vi "DoGetNewUser.vi"(8 "error in (no error)":errorcluster, 9 "LastUserName":string, 10 "IsInitialLogin":bool, 11 "Sequence Context In":refnum<k7>) -> (0 "error out":errorcluster, 1 "LoginName":string, 2 "isValidUser":bool, 3 "Sequence Context Out":refnum<k7>, 5 "logOut":bool)   [LabVIEW 2021]
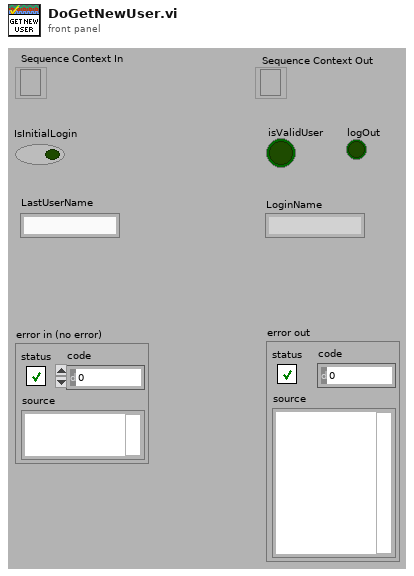
[diagram p1: front panel]
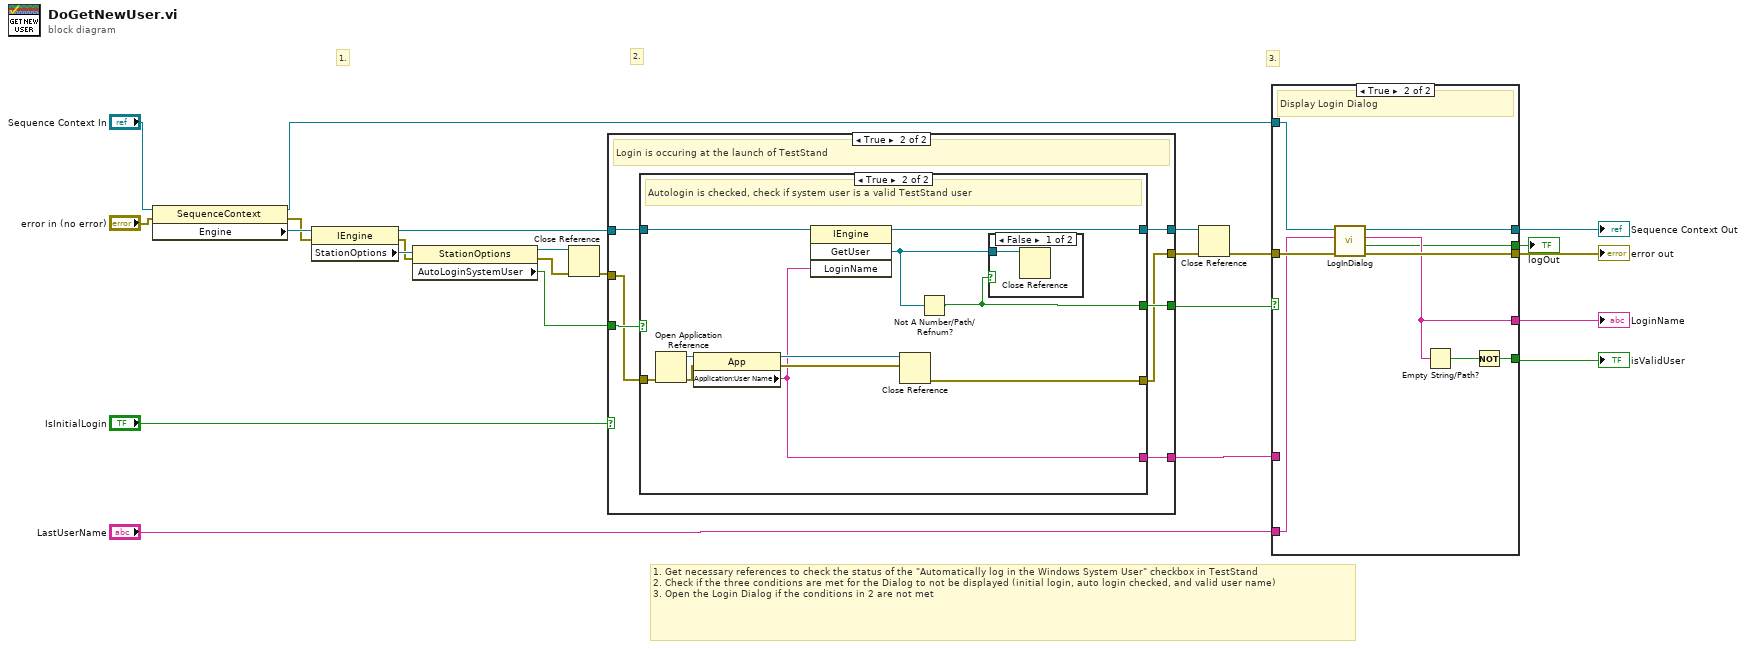
[diagram p0: block diagram]
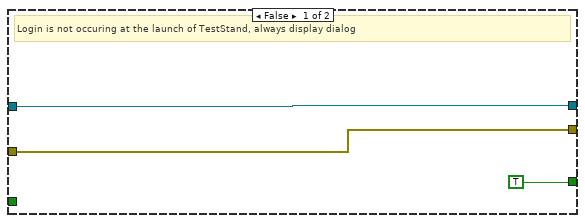
[diagram p2: hidden frame]
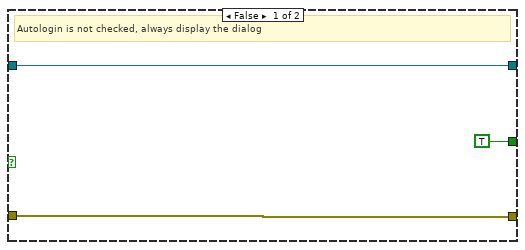
[diagram p3: hidden frame]
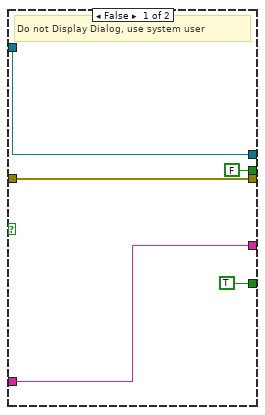
[diagram p5: hidden frame]
diagram:
  # "1. Get necessary references to check the status of the \"Automatically log in the Windows System User\" checkbox in TestStand\n2. Check if the three conditions are met for the Dialog to not be displayed (initial login, auto login checked, and valid user name)\n3. Open the Login Dialog if the conditions in 2 are not met"
  # "3."
  # "2."
  # "1."
  n1 = property class="SequenceContext"(reference="Sequence Context In", error in="error in (no error)") -> (reference out=w11:refnum<k7>, error out=w3:errorcluster, "Engine"=w17:refnum<k7>)
  n2 = property class="IEngine"(reference=w17, error in=w3) -> (reference out=w21:refnum<k7>, error out=w20:errorcluster, "StationOptions"=w24:refnum<k7>)
  n3 = property class="StationOptions"(reference=w24, error in=w20) -> (reference out=w16:refnum<k7>, error out=w14:errorcluster, "AutoLoginSystemUser"=w22:bool)
  n4 = Close Reference(reference=w16, error in (no error)=w14) -> (error out=w15:errorcluster)
  n5 = case shown="True" "IsInitialLogin" {
    tunnel: w22 -> [_ w34]
    tunnel: [TRUE ("displayLoginDialog") w33] -> w18
    tunnel: w21 -> [w25 w30]
    tunnel: [w26 w31] -> w9
    tunnel: w15 -> [w26 w32]
    tunnel: [w25 w29] -> w7
    tunnel: [_ w28] -> w2
    frame False {
      # "Login is not occuring at the launch of TestStand, always display dialog"
    }
    frame True {
      # "Login is occuring at the launch of TestStand"
      n6 = case shown="True" w34 {
        tunnel: [TRUE ("displayLoginDialog") w38] -> w33
        tunnel: w32 -> [w36 w48]
        tunnel: [w36 w45] -> w31
        tunnel: w30 -> [w35 w42]
        tunnel: [w35 w41] -> w29
        tunnel: [_ w40] -> w28
        frame False {
          # "Autologin is not checked, always display the dialog"
        }
        frame True {
          # "Autologin is checked, check if system user is a valid TestStand user"
          n7 = Open Application Reference(8:w48) -> (0:w46:errorcluster, 3:w47:refnum<vi>)  [unwired: 3 in]
          n8 = property class="App"(reference=w47, error in=w46) -> (reference out=w44:refnum<vi>, error out=w43:errorcluster, "Application:User Name"=w40:string)
          n9 = invoke class="IEngine" method="GetUser"(reference=w42, "LoginName"=w40) -> (reference out=w41:refnum<k7>, "GetUser"=w39:refnum<k7>)  [unwired: 2 in, 2 out]
          n10 = Close Reference(reference=w44, error in (no error)=w43) -> (error out=w45:errorcluster)
          n11 = Not A Number/Path/Refnum?(number/path/refnum=w39) -> (NaN/Path/Refnum?=w38:bool)
          n12 = case shown="False" w38 {
            tunnel: w39 -> [w49 _]
            frame False {
              n13 = Close Reference(reference=w49) -> ()  [unwired: 1 in, 1 out]
            }
            frame True {
            }
          }
        }
      }
    }
  }
  n14 = Close Reference(reference=w7, error in (no error)=w9) -> (error out=w8:errorcluster)
  n15 = case shown="True" w18 {
    tunnel: [w52 w61] -> w6
    tunnel: [TRUE ("HasPrivilege") w56] -> w19
    tunnel: [w51 w58] -> w10
    tunnel: "LastUserName" -> [_ w59]
    tunnel: w11 -> [w53 w63]
    tunnel: [w53 w62] -> w12
    tunnel: w8 -> [w52 w60]
    tunnel: w2 -> [w51 _]
    tunnel: [FALSE ("logOut") w55] -> w1
    frame False {
      # "Do not Display Dialog, use system user"
    }
    frame True {
      # "Display Login Dialog"
      n16 = call "LogInDialog.vi"("error in (no error)"=w60, "Default User"=w59, "Sequence Context In"=w63) -> ("error out"=w61:errorcluster, "Continue?"=w55:bool, "UserName"=w58:string, "Sequence Context Out"=w62:refnum<k7>)  [unwired: 5 in]
      n17 = Empty String/Path?(string/path=w58) -> (empty?=w57:bool)
      n18 = Not(x=w57) -> (.not. x?=w56:bool)
    }
  }
  "error out" <- w6
  "isValidUser" <- w19
  "LoginName" <- w10
  "Sequence Context Out" <- w12
  "logOut" <- w1
